vi "Right Motor Set Power.vi"(8 "error in":errorcluster, 10 "Disable Ramp":bool, 11 "Output":dbl) -> (0 "error out":errorcluster)   [LabVIEW 2015]
uses:
  Support/Global Objects.vi
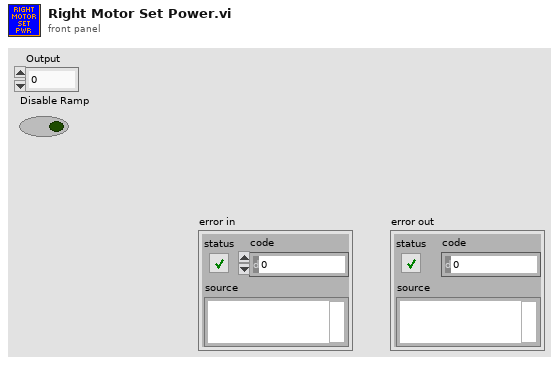
[diagram p1: front panel]
types:
  T1 = typedef "2 Motor Typedef.ctl" = cluster{"Motor1":T2, "Motor2":T2, "Last Motor Power":dbl}
  T2 = typedef "WPI_MotorControlDeviceRef.ctl" = cluster{"DeviceStatus":errorcluster, "Type":T3, "PWM":cluster{"PWM Channel":T4, "DeadBand":T5}, "CAN":cluster{"Device Number":u8, "Control Mode":T6, "Semaphore":T7, "Max Vout":dbl, "TalonSRX Control Mode":T8}, "Invert":bool}
  T3 = typedef "WPI_MotorControlType.ctl" = enum16{"PWM", "CAN", "CANTalonSRX"}
  T4 = typedef "FPGA_DIOPWMChannel.ctl" = enum8{"PWM 0", "PWM 1", "PWM 2", "PWM 3", "PWM 4", "PWM 5", "PWM 6", "PWM 7", "PWM 8", "PWM 9", "PWM MXP 0", "PWM MXP 1", "PWM MXP 2", "PWM MXP 3", "PWM MXP 4", "PWM MXP 5", "PWM MXP 6", "PWM MXP 7", "PWM MXP 8", "PWM MXP 9", "Invalid"}
  T5 = typedef "WPI_PWMDeadband.ctl" = cluster{"Name":string, "maxPositivePwm":i32, "minPositivePwm":i32, "centerPwm":i32, "maxNegativePwm":i32, "minNegativePwm":i32, "angularRange":u16}
  T6 = typedef "WPI_CANJaguar_ControlMode.ctl" = enum8{"Percent VBus", "Current", "Speed", "Position", "Voltage"}
  T7 = typedef "Semaphore RefNum" = refnum<k1>
  T8 = typedef "WPI_CANTalonSRX_APIControlMode.ctl" = enum8{"Percent VBus", "Speed", "Position", "Slave", "Unchanged / Invalid", "Voltage Compensation", "Current", "Motion Profile"}
  T9 = typedef "Configuration.ctl" = cluster{"Throttle Dead Zone":dbl, "Throttle Ramp Rate":dbl, "Turn Dead Zone":dbl, "Auton":cluster{"Motion Plan P":dbl, "Motion Plan I":dbl, "Motion Plan D":dbl}, "Auto Upshift Enabled":bool, "Upshift Min Throttle":dbl, "Upshift Min Velocity":dbl, "Min time before upshift":dbl, "Shift Throttle Detent":u32, "Min time before downshift":dbl, "Turn PID":cluster{"Motion Plan P":dbl, "Motion Plan I":dbl, "Motion Plan D":dbl}, "Auto Coast Downshift":bool, "Downshift Coast Max Vel":dbl, "Downshift Coast Throttle Epsilon":dbl, "Left Motor Calibration":dbl, "Right Motor Calibration":dbl}
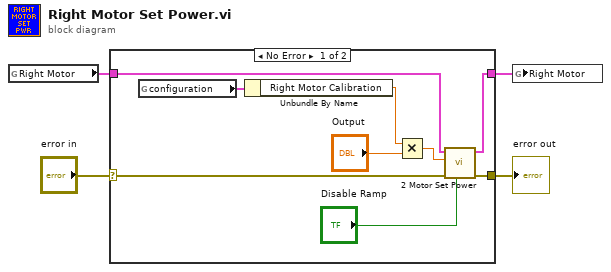
[diagram p0: block diagram]
diagram:
  n1 = global read "Global Objects.vi" "Right Motor"() -> (w2:T1)
  n2 = case shown="No Error" "error in" {
    selector: "error in" -> [w11 w15]
    tunnel: [w10 w15] -> w3
    tunnel: w2 -> [w13 w14]
    tunnel: [w12 w14] -> w1
    frame No Error {
      n3 = global read "Global Objects.vi" "configuration"() -> (w6:T9)
      n4 = Unbundle By Name(w6) -> ("Right Motor Calibration"=w5:dbl)
      n5 = Multiply(x=w5, y="Output") -> (x*y=w7:dbl)
      n6 = call "2 Motor Set Power.vi"("Disable Ramp"="Disable Ramp", "error in"=w11, "Output"=w7, "Motor In"=w13) -> ("error out"=w10:errorcluster, "Motor Out"=w12:T1)  [unwired: 6 in]
    }
    frame Error {
    }
  }
  "error out" <- w3
  n7 = global write "Global Objects.vi" "Right Motor"(w1) -> ()
